vi "Connect with Pad.vi"(8 "error in (no error)":errorcluster) -> (0 "error out":errorcluster, 3 "device ID":refnum<k1>, 5 "Connected?":bool)   [LabVIEW 2014]
uses:
  <vilib>/Utility/error.llb/DialogType.ctl
  <vilib>/Utility/inputDevices.llb/closeJoystick.vi
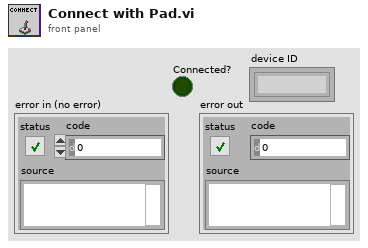
[diagram p1: front panel]
types:
  T1 = cluster{"axes total":u32, "buttons total":u32, "pov total":u32, "device name":string}[]
  T2 = typedef "DialogType.ctl" = u16
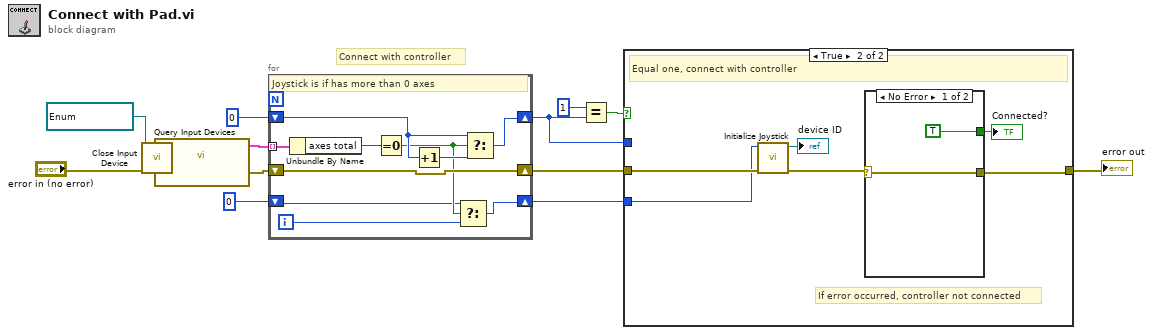
[diagram p0: block diagram]
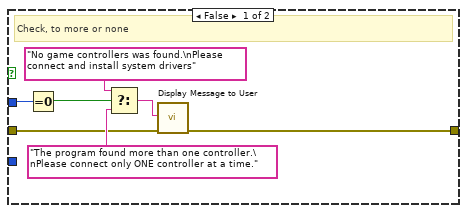
[diagram p2: hidden frame]
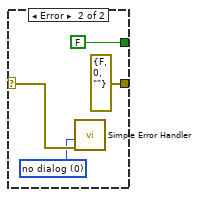
[diagram p3: hidden frame]
diagram:
  w1 = refnum<k1> refnum items=["JOYSTICK"] ("device ID")
  # "Connect with controller"
  n1 = call-poly <vilib>:"Close Input Device.vi"("error in (no error)"="error in (no error)", "device ID"=w1) -> ("error out"=w7:errorcluster)  [unwired: 8 in]
  n2 = call <vilib>:"Query Input Devices.vi"("error in (no error)"=w7) -> ("error out"=w4:errorcluster, "joystick info"=w5:T1)  [unwired: 7 in, 2 out]
  n3 = for {
    shift-right: [w18] -> w11
    shift-left: w4 -> [w18]
    tunnel: w5 -> [w23] mode=indexing
    shift-right: [w21] -> w13
    shift-left: 0 -> [w20]
    shift-right: [w15] -> w2
    shift-left: 0 -> [w16]
    i -> [w14]
    # "Joystick is if has more than 0 axes"
    n4 = Unbundle By Name(w23) -> ("axes total"=w22:u32)
    n5 = Equal To 0?(x=w22) -> (x = 0?=w17:bool)
    n6 = Increment(x=w20) -> (x+1=w19:i32)
    n7 = Select(t=w16, s=w17, f=w14) -> (s? t:f=w15:i32)
    n8 = Select(t=w20, s=w17, f=w19) -> (s? t:f=w21:i32)
  }
  n9 = Equal?(x=1, y=w13) -> (x = y?=w10:bool)
  n10 = case shown="True" w10 {
    tunnel: w11 -> [w26 w36]
    tunnel: [w25 w33] -> w12
    tunnel: w13 -> [w30 _]
    tunnel: w2 -> [_ w31]
    frame False {
      # "Check, to more or none"
      n11 = Equal To 0?(x=w30) -> (x = 0?=w29:bool)
      n12 = Select(t="No game controllers was found.\nPlease connect and install system drivers", s=w29, f="The program found more than one controller.\nPlease connect only ONE controller at a time.") -> (s? t:f=w24:string)
      n13 = call "Display Message to User"("error in (no error)"=w26, "Message"=w24) -> ("error out"=w25:errorcluster)  [unwired: 8 in, 1 out]
    }
    frame True {
      # "If error occurred, controller not connected"
      # "Equal one, connect with controller"
      n14 = call <vilib>:"Initialize Joystick.vi"("error in (no error)"=w36, "device index"=w31) -> ("error out"=w34:errorcluster, "device ID"=→"device ID":refnum<k1>)  [unwired: 8 in]
      n15 = case shown="No Error" w34 {
        selector: w34 -> [w38 w41]
        tunnel: [w38 errorcluster {"status"=FALSE, "code"=0, "source"=""} ("error IO")] -> w33
        tunnel: [TRUE FALSE] -> w32
        frame No Error {
        }
        frame Error {
          w40 = T2 0 items=["no dialog", "OK message", "continue or stop message", "OK message + warnings", "continue/stop + warnings"] ("type of dialog (OK msg:1)")
          n16 = call <vilib>:"Simple Error Handler.vi"("type of dialog (OK msg:1)"=w40, "error in (no error)"=w41) -> ()  [unwired: 3 in, 5 out]
        }
      }
      "Connected?" <- w32
    }
  }
  "error out" <- w12
